vi "Arduino single device test Feb 2017.vi"() -> ()   [LabVIEW 2014]
uses:
  <vilib>/Analysis/baseanly.llb/Mean (DBL).vi
  <vilib>/Instr/_visa.llb/VISA Configure Serial Port (Instr).vi
  <vilib>/Utility/file.llb/Write To Spreadsheet File (string).vi
  <vilib>/Analysis/NI_AALBase.lvlib
panel:
  in  "Arduino address":refnum<visa-resource-name>
  out "Measurements":T1 {"Frequency (Hz)" format="%#_12g"}
  out "Save file path":path
  in  "Save data?":bool
  out "Waveform Chart":dbl(graph)
  in  "Cluster":T2
  in  "Stop Button":bool
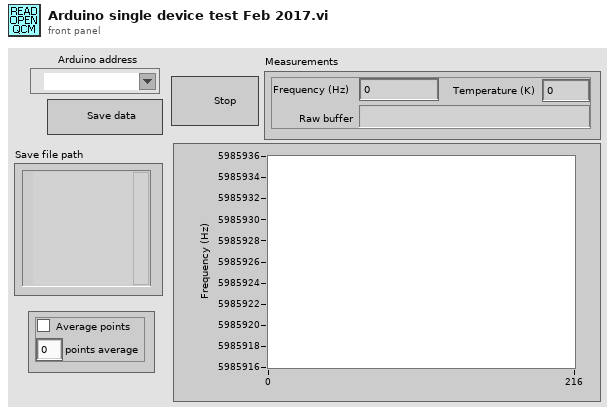
[diagram p1: front panel]
types:
  T1 = cluster{"Frequency (Hz)":dbl, "Temperature (K)":dbl, "Raw buffer":string}
  T2 = cluster{"points average":i32, "average points?":bool}
  T3 = enum16{"open", "replace", "create", "open or create", "replace or create", "replace or create with confirmation"}
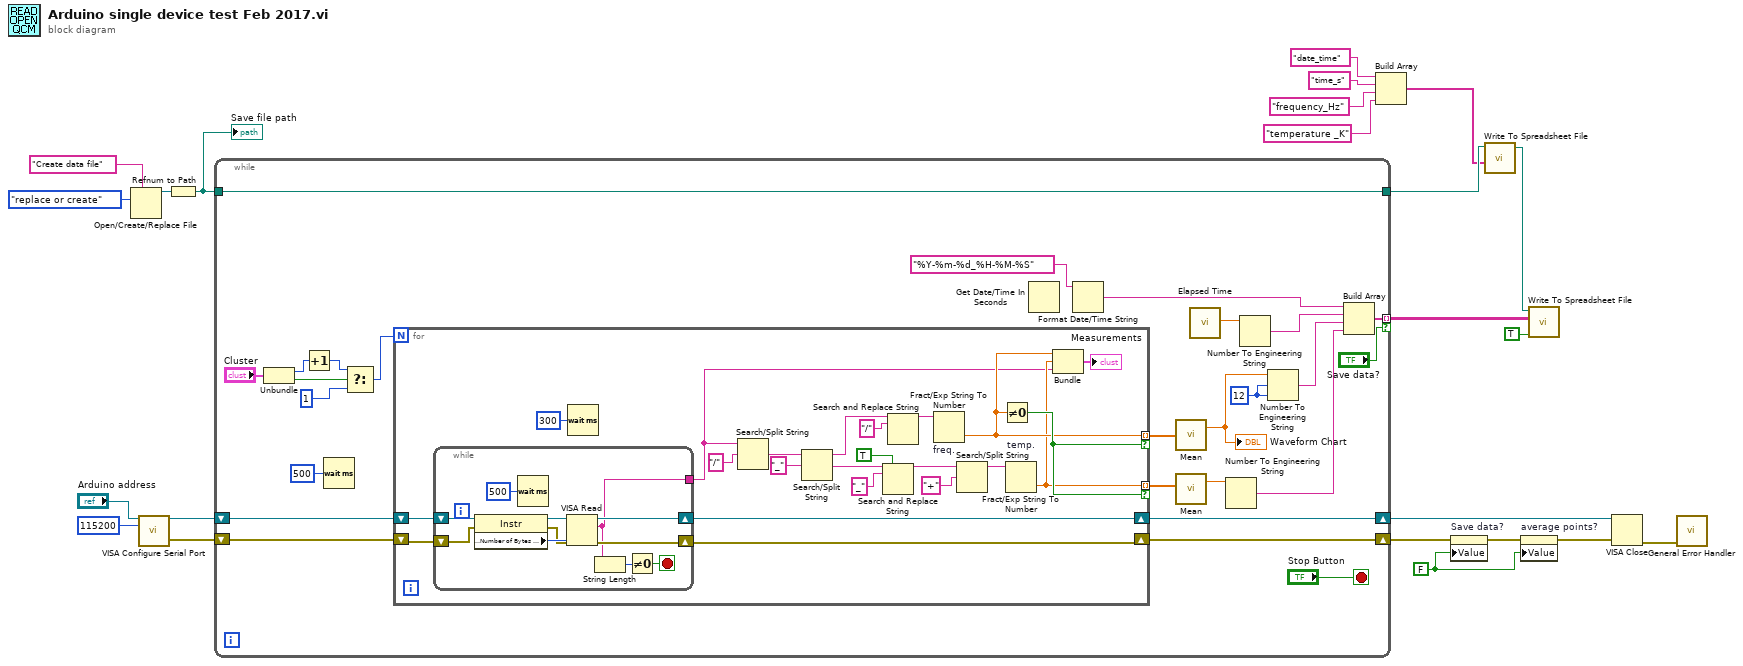
[diagram p0: block diagram]
diagram:
  w5 = FALSE ("Save data?")
  n1 = Open/Create/Replace File(prompt="Create data file", operation (0:open)=T3."replace or create") -> (refnum out=w13:refnum<file>)  [unwired: 4 in, 2 out]
  n2 = call-poly "VISA Configure Serial Port"("VISA resource name"="Arduino address", "baud rate (9600)"=u32 115200) -> ("VISA resource name out"=w21:refnum<visa-resource-name>, "error out"=w20:errorcluster)  [unwired: 12 in]
  n3 = Refnum to Path(1:w13) -> (0:w3:path)
  "Save file path" <- w3
  n4 = while {
    shift-right: [w49] -> w22
    shift-left: w21 -> [w47]
    shift-right: [w48] -> w7
    shift-left: w20 -> [w46]
    tunnel: [w33] -> w19 mode=indexing if="Save data?"
    tunnel: [w32] -> w16
    tunnel: w3 -> [w32]
    stop <- "Stop Button" stop-if-true
    w41 = 12 ("offset")
    n5 = Unbundle("Cluster") -> ("points average"=w27:i32, "average points?"=w24:bool)
    n6 = Increment(x=w27) -> (x+1=w25:i32)
    n7 = Wait (ms)(milliseconds to wait=u32 500) -> ()  [unwired: 1 out]
    n8 = Select(t=w25, s=w24, f=1) -> (s? t:f=w35:i32)
    n9 = for {
      N: w35 -> [_]
      tunnel: [w55] -> w43 mode=indexing if=w56
      shift-right: [w51] -> w49
      shift-left: w47 -> [w59]
      shift-right: [w50] -> w48
      shift-left: w46 -> [w58]
      tunnel: [w54] -> w30 mode=indexing if=w56
      n10 = while {
        shift-right: [w78] -> w51
        shift-left: w59 -> [w82]
        shift-right: [w73] -> w50
        shift-left: w58 -> [w81]
        tunnel: [w72] -> w52
        stop <- w76 stop-if-true
        # "wait until bytes are ready"
        n11 = property class="Instr"(reference=w82, error in=w81) -> (reference out=w79:refnum<visa-resource-name>, error out=w74:errorcluster, "Serial Settings:Number of Bytes at Serial Port"=w77:u32)
        n12 = Wait (ms)(milliseconds to wait=u32 500) -> ()  [unwired: 1 out]
        n13 = VISA Read(VISA resource name=w79, byte count=w77, error in (no error)=w74) -> (VISA resource name out=w78:refnum<visa-resource-name>, read buffer=w72:string, error out=w73:errorcluster)  [unwired: 1 out]
        n14 = String Length(string=w72) -> (length=w75:i32)
        n15 = Not Equal To 0?(x=w75) -> (x != 0?=w76:bool)
      }
      n16 = Wait (ms)(milliseconds to wait=u32 300) -> ()  [unwired: 1 out]
      n17 = Search/Split String(string=w52, search string/char (-)="/") -> (match + rest of string=w65:string)  [unwired: 1 in, 2 out]
      n18 = Search/Split String(string=w65, search string/char (-)="_") -> (substring before match=w71:string, match + rest of string=w66:string)  [unwired: 1 in, 1 out]
      n19 = Search and Replace String(replace all?=TRUE ("replace all? (F)"), input string=w66, search string="_") -> (result string=w60:string)  [unwired: 5 in, 3 out]
      n20 = Search and Replace String(input string=w71, search string="/" ("replace string (\"\")")) -> (result string=w62:string)  [unwired: 6 in, 3 out]
      n21 = Fract/Exp String To Number "freq."(string=w62) -> (number=w55:dbl)  [unwired: 3 in, 1 out]
      n22 = Search/Split String(string=w60, search string/char (-)="+") -> (substring before match=w69:string)  [unwired: 1 in, 2 out]
      n23 = Not Equal To 0?(x=w55) -> (x != 0?=w56:bool)
      n24 = Fract/Exp String To Number "temp."(string=w69) -> (number=w54:dbl)  [unwired: 3 in, 1 out]
      n25 = Bundle(w55, w54, "read buffer"=w52) -> (→"Measurements":cluster{dbl, dbl, "read buffer":string})  [unwired: 1 in]
    }
    n26 = Get Date/Time In Seconds() -> ()  [unwired: 1 out]
    n27 = Format Date/Time String(time format string (%c)="%Y-%m-%d_%H-%M-%S") -> (date/time string=w39:string)  [unwired: 2 in]
    n28 = call-poly <vilib>:"Mean.vi"("X"=w43) -> ("mean"=w37:dbl)  [unwired: 1 out]
    "Waveform Chart" <- w37
    n29 = call-poly <vilib>:"Mean.vi"("X"=w30) -> ("mean"=w29:dbl)  [unwired: 1 out]
    n30 = call "Elapsed Time"() -> ("Elapsed Time (s)"=w40:dbl)  [unwired: 12 in, 7 out]
    n31 = Number To Engineering String(4:w29) -> (0:w28:string)  [unwired: 3 in]
    n32 = Number To Engineering String(4:w40) -> (0:w38:string)  [unwired: 3 in]
    n33 = Number To Engineering String(2:w41, 3:w41, 4:w37) -> (0:w36:string)  [unwired: 1 in]
    n34 = Build Array(w39, w38, w36, w28) -> (w33:string[])
  }
  n35 = Build Array("date_time" ("time format string (%c)"), "time_s" ("time format string (%c)"), "frequency_Hz" ("time format string (%c)"), "temperature _K" ("time format string (%c)")) -> (w15:string[])
  n36 = property on="Save data?" class="Bool (strict)"(error in=w7, "Value"=w5) -> (error out=w8:errorcluster)  [unwired: 1 in, 1 out]
  n37 = call-poly <vilib>:"Write To Spreadsheet File.vi"("1D data"=w15, "file path (dialog if empty)"=w16) -> ("new file path (Not A Path if cancelled)"=w18:path)  [unwired: 6 in]
  n38 = property on="average points?" class="Bool (strict)"(error in=w8, "Value"=w5) -> (error out=w6:errorcluster)  [unwired: 1 in, 1 out]
  n39 = call-poly <vilib>:"Write To Spreadsheet File.vi"("append to file? (new file:F)"=TRUE, "2D data"=w19, "file path (dialog if empty)"=w18) -> ()  [unwired: 5 in, 1 out]
  n40 = VISA Close(VISA resource name=w22, error in (no error)=w6) -> (error out=w4:errorcluster)
  n41 = call <vilib>:"General Error Handler.vi"("error in (no error)"=w4) -> ()  [unwired: 10 in, 5 out]
